vi "Write Reset.vi"(8 "error in (no error)":errorcluster, 10 "Reset":bool, 11 "Reset Device Msg in":refnum<class "Reset Device Msg.lvclass">) -> (0 "error out":errorcluster, 3 "Reset Device Msg out":refnum<class "Reset Device Msg.lvclass">)   [LabVIEW 2016, in "CS++DeviceActor.lvlib" / "Reset Device Msg.lvclass"]
uses:
  Reset Device Msg.lvclass
  Reset Device Msg.lvclass/Reset Device Msg.ctl
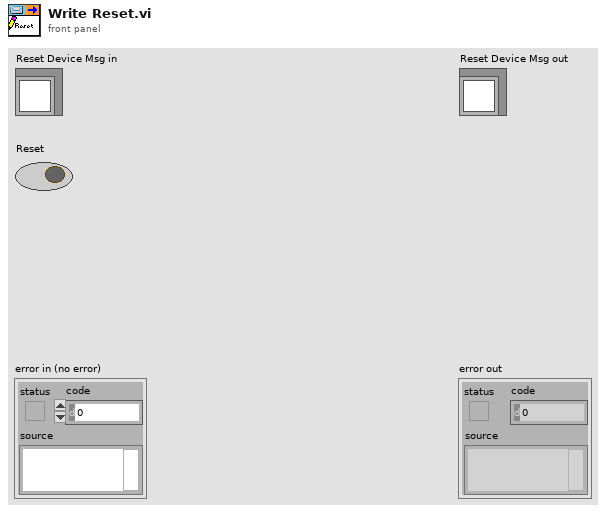
[diagram p1: front panel]
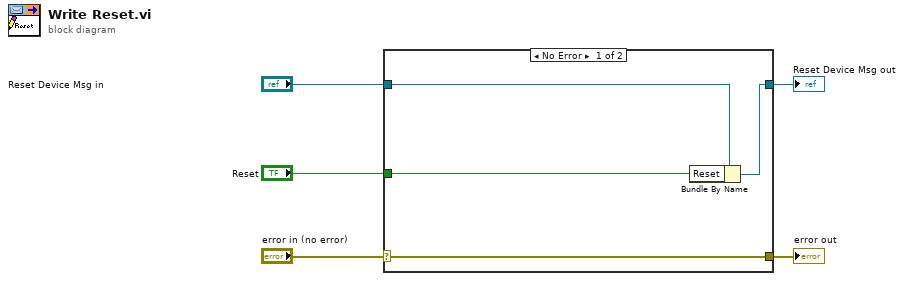
[diagram p0: block diagram]
diagram:
  n1 = case shown="No Error" "error in (no error)" {
    selector: "error in (no error)" -> [w9 w10]
    tunnel: [w9 w10] -> w4
    tunnel: [w7 w11] -> w2
    tunnel: "Reset Device Msg in" -> [w8 w11]
    tunnel: "Reset" -> [w6 _]
    frame No Error {
      n2 = Bundle By Name(cluster=w8, "Reset"=w6) -> (w7:refnum<class "Reset Device Msg.lvclass">)
    }
    frame Error {
    }
  }
  "error out" <- w4
  "Reset Device Msg out" <- w2
